vi "Get VI RefNum.vi"(8 "error in (no error)":errorcluster, 11 "VI Ref":refnum<vi>) -> (0 "error out":errorcluster, 2 "window refnum":T1, 3 "VI Ref out":refnum<vi>)   [LabVIEW 2020, in "MacroAssert.lvlib" / "Win Util.lvlib"]
uses:
  Win Util.lvlib
  Window Refnum.ctl
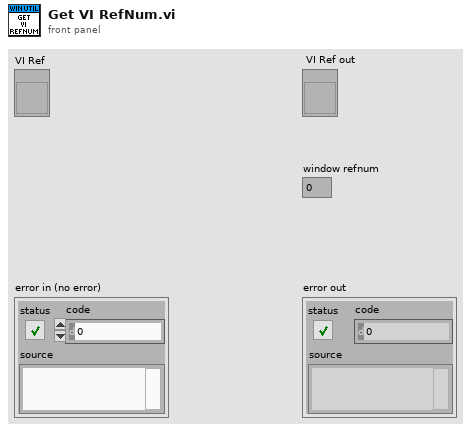
[diagram p1: front panel]
types:
  T1 = typedef "MacroAssert.lvlib/Win Util.lvlib/Window Refnum.ctl" = u64
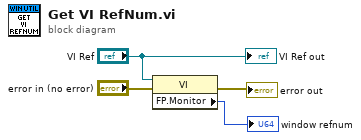
[diagram p0: block diagram]
diagram:
  n1 = property class="VI"(reference="VI Ref", error in="error in (no error)") -> (error out=→"error out":errorcluster, "FP.Monitor"=→"window refnum":u16)  [unwired: 1 out]
  "VI Ref out" <- "VI Ref"
